vi "Global Offsets.vi"() -> ()   [LabVIEW 2019]
panel:
  in  "Offsets":dbl[](array[numeric]) format="%.3f"
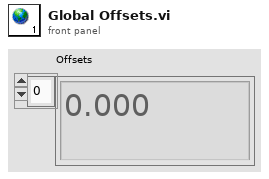
[diagram p1: front panel]
diagram:
